vi "Measure.vi"(8 "error in (no error)":errorcluster, 9 "measurement configuration":variant, 10 "measure call context in":refnum<class "Measure Call Context.lvclass">, 11 "measurement plugin in":refnum<class "FPT Framework.lvclass">) -> (0 "error out":errorcluster, 1 "measurement results":variant, 2 "measure call context out":refnum<class "Measure Call Context.lvclass">, 3 "measurement plugin out":refnum<class "FPT Framework.lvclass">)   [LabVIEW 2023, in "FPT Framework.lvclass"]
uses:
  FPT Framework.lvclass
  <vilib>/Plug-In SDKs/Measurements/Measure Call Context/Measure Call Context.lvclass
  Measurement Configuration.ctl
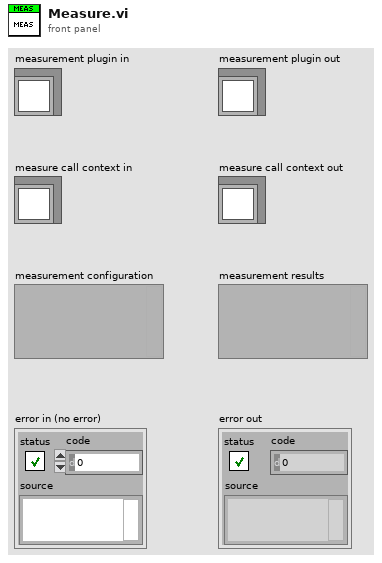
[diagram p1: front panel]
types:
  T1 = typedef "FPT Framework.lvclass/Measurement Configuration.ctl" = cluster{"Automation Test":bool, "Power sequencing file path":string, "SMU name":string, "SMU channel":string, "Compression_Expected DUT Gain (dB)":dbl, "Compression_Max Linear Range (dBm)":dbl, "Compression_Compression Point (dB)":dbl, "Compression_Target Pin (dBm)":dbl, "Compression_RFSG Frequency Start (Hz)":dbl, "Compression_RFSG Frequency Stop (Hz)":dbl, "Compression_RFSG Number of Frequency Step":i32, "Compression_RFSG Power Start (dBm)":dbl, "Compression_RFSG Power Stop(dBm)":dbl, "Compression_RFSG Power Step Size (dB)":dbl, "Compression_RBW (Hz)":dbl}
  T2 = typedef "FPT Framework.lvclass/Measurement Results.ctl" = cluster{"Status":string, "per Freq Plot Names":string[], "Linear Gain vs Freq":dbl[][], "OPxdB vs Freq":dbl[][], "Pout@Pin vs Freq":dbl[][], "Gain@Pin vs Freq":dbl[][], "PAE@Pin vs Freq":dbl[][], "Pout vs Pin per Freq":dbl[][], "Gain vs Pin per Freq":dbl[][], "PAE vs Pin per Freq":dbl[][], "Pout@Pin (Mean)":dbl, "Gain@Pin (Mean)":dbl, "PAE@Pin (Mean)":dbl, "Linear Gain (Mean)":dbl, "OPxdB (Mean)":dbl}
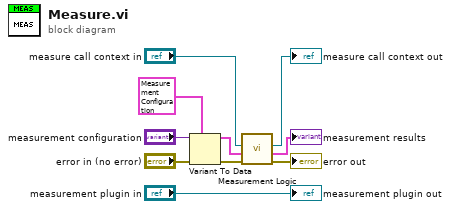
[diagram p0: block diagram]
diagram:
  n1 = Variant To Data(error in="error in (no error)", type=T1 {"Automation Test"=FALSE, "Power sequencing file path"="", "SMU name"="", "SMU channel"="", "Compression_Expected DUT Gain (dB)"=17.5, "Compression_Max Linear Range (dBm)"=-10.0, "Compression_Compression Point (dB)"=1.0, "Compression_Target Pin (dBm)"=1.0, "Compression_RFSG Frequency Start (Hz)"=6000000000.0, "Compression_RFSG Frequency Stop (Hz)"=18000000000.0, "Compression_RFSG Number of Frequency Step"=11, "Compression_RFSG Power Start (dBm)"=-20.0, "Compression_RFSG Power Stop(dBm)"=4.0, "Compression_RFSG Power Step Size (dB)"=1.0, "Compression_RBW (Hz)"=5000000.0} ("measurement configuration"), Variant="measurement configuration") -> (data=w1:T1, error out=w7:errorcluster)
  n2 = call "Measurement Logic.vi"("error in"=w7, "measurement configuration"=w1, "measure call context in"="measure call context in") -> ("error out"=→"error out":errorcluster, "measurement results"=→"measurement results":T2, "measure call context out"=→"measure call context out":refnum<class "Measure Call Context.lvclass">)  [unwired: 6 in]
  "measurement plugin out" <- "measurement plugin in"
